vi "Digital_write_PFI_trigger.vi"() -> ()   [LabVIEW 2020]
uses:
  <vilib>/DAQmx/write.llb/DAQmx Write (Digital Wfm 1Chan NSamp).vi
  <vilib>/DAQmx/create/channels.llb/DAQmx Create Channel (DO-Digital Output).vi
  <vilib>/DAQmx/configure/timing.llb/DAQmx Timing (Sample Clock).vi
  <vilib>/Waveform/DWDTOps.llb/Digital Pattern Generator (Marching Values).vi
  <vilib>/Waveform/DWDTOps.llb/DWDT Uncompress Digital.vi
  <vilib>/DAQmx/miscellaneous.llb/DAQmx Fill In Error Info.vi
panel:
  in  "Y":digitaldata
  out "Digital Waveform Graph 2":digitalwaveform(graph)
  out "Digital Waveform Graph":digitalwaveform(graph)
  in  "samples per channel":i32=1000
  in  "rate":dbl=1000.0 format="%0.2f"
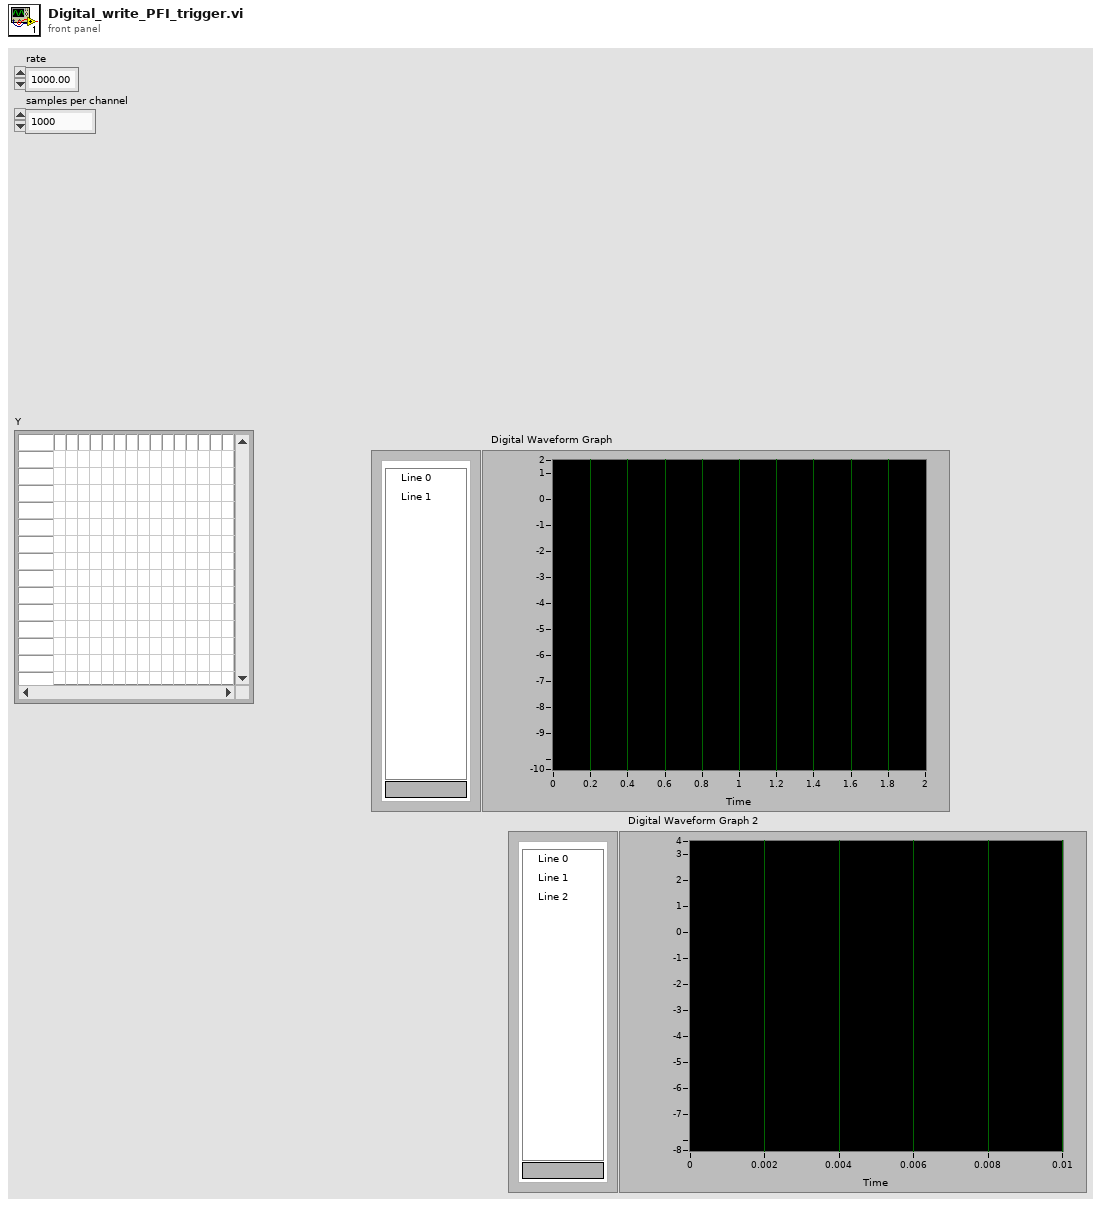
[diagram p1: front panel]
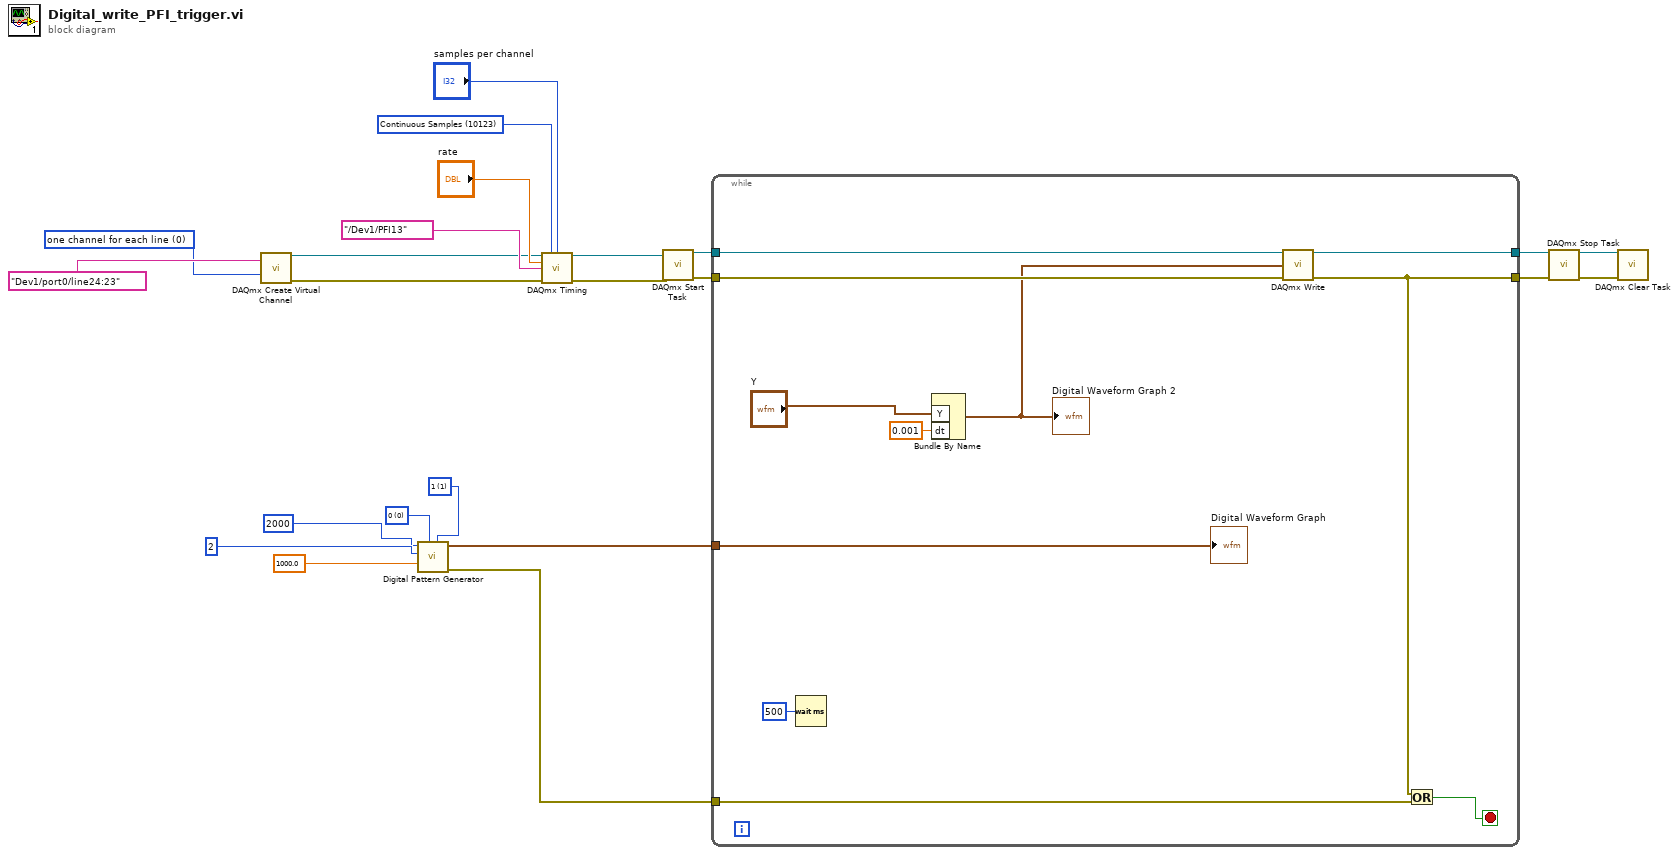
[diagram p0: block diagram]
diagram:
  w7 = u8 1 items=["0", "1", "Z", "L", "H", "X", "T", "V"] ("marching value")
  w6 = u8 0 items=["0", "1", "Z", "L", "H", "X", "T", "V"] ("value")
  w13 = 10123 items=["Finite Samples"=10178, "Continuous Samples"=10123, "Hardware Timed Single Point"=12522] ("sample mode")
  w16 = 0 items=["one channel for each line", "one channel for all lines"] ("line grouping")
  n1 = call-poly <vilib>:"DAQmx Create Virtual Channel.vi"("lines"=tag "Dev1/port0/line24:23", "line grouping"=w16) -> ("task out"=w11:refnum<k21>, "error out"=w10:errorcluster)  [unwired: 12 in]
  n2 = call-poly <vilib>:"Digital Pattern Generator.vi"("marching value"=w7, "hold value"=w6, "sample rate"=1000.0, "number of signals"=u32 2, "number of samples"=u32 2000) -> ("error out"=w2:errorcluster, "digital waveform"=w1:digitalwaveform)  [unwired: 5 in]
  n3 = call-poly <vilib>:"DAQmx Timing.vi"("task/channels in"=w11, "sample mode"=w13, "samples per channel"="samples per channel", "rate"="rate", "source"=tag "/Dev1/PFI13", "error in"=w10) -> ("task out"=w9:refnum<k21>, "error out"=w8:errorcluster)  [unwired: 8 in]
  n4 = call <vilib>:"DAQmx Start Task.vi"("task/channels in"=w9, "error in"=w8) -> ("task out"=w23:refnum<k21>, "error out"=w22:errorcluster)  [unwired: 12 in]
  n5 = while {
    tunnel: w23 -> [w34]
    tunnel: w22 -> [w33]
    tunnel: [w32] -> w21
    tunnel: [w30] -> w20
    tunnel: w2 -> [w27]
    tunnel: w1 -> [w26]
    stop <- w31 stop-if-true
    n6 = Wait (ms)(milliseconds to wait=u32 500) -> ()  [unwired: 1 out]
    n7 = Bundle By Name("Y"="Y", "dt"=0.001) -> (w24:digitalwaveform)  [unwired: 1 in]
    "Digital Waveform Graph 2" <- w24
    n8 = call-poly <vilib>:"DAQmx Write.vi"("task/channels in"=w34, "data"=w24, "error in"=w33) -> ("task out"=w32:refnum<k21>, "error out"=w30:errorcluster)  [unwired: 10 in, 1 out]
    n9 = Or(x=w30, y=w27) -> (x .or. y?=w31:bool)
    "Digital Waveform Graph" <- w26
  }
  n10 = call <vilib>:"DAQmx Stop Task.vi"("task/channels in"=w21, "error in"=w20) -> ("task out"=w19:refnum<k21>, "error out"=w18:errorcluster)  [unwired: 12 in]
  n11 = call <vilib>:"DAQmx Clear Task.vi"("task in"=w19, "error in"=w18) -> ()  [unwired: 13 in, 1 out]
